vi "test-pose3d.vi"(8 "error in (no error)":errorcluster) -> (0 "error out":errorcluster, 3 "All PASSED":bool)   [LabVIEW 2019]
uses:
  <vilib>/Rock Robotics/WPI/ThirdParty/JAS_Junk/TrajLib/Rotation2d_CreateAngle.vi
  <vilib>/Rock Robotics/WPI/ThirdParty/JAS_Junk/TrajLib/Translation2d_Create.vi
  <vilib>/Rock Robotics/WPI/ThirdParty/JAS_Junk/TrajLib/Quaternion_New.vi
  <vilib>/Rock Robotics/WPI/ThirdParty/JAS_Junk/TrajLib/Pose3d_getTranslation3d.vi
  <vilib>/Rock Robotics/WPI/ThirdParty/JAS_Junk/TrajLib/Translation3d_ToTranslation2d.vi
  <vilib>/Rock Robotics/WPI/ThirdParty/JAS_Junk/TrajLib/Rotation3d_ToRotation2d.vi
  <vilib>/Rock Robotics/WPI/ThirdParty/JAS_Junk/TrajLib/Pose2d_New_TRRO.vi
  <vilib>/Rock Robotics/WPI/ThirdParty/JAS_Junk/TrajLib/Translation2d_Equals.vi
  <vilib>/Rock Robotics/WPI/ThirdParty/JAS_Junk/TrajLib/Rotation2d_Equals.vi
  <vilib>/Rock Robotics/WPI/ThirdParty/JAS_Junk/TrajLib/Matrix_NormF.vi
  <vilib>/Rock Robotics/WPI/ThirdParty/JAS_Junk/TrajLib/Rotation3d_Create_Default.vi
  <vilib>/Rock Robotics/WPI/ThirdParty/JAS_Junk/TrajLib/Quaternion_Get_All.vi
  <vilib>/Rock Robotics/WPI/ThirdParty/JAS_Junk/TrajLib/Rotation3d_GetQuaterion.vi
  <vilib>/Rock Robotics/WPI/ThirdParty/JAS_Junk/TrajLib/Transform3d_GetTranslation3d.vi
  <vilib>/Rock Robotics/WPI/ThirdParty/JAS_Junk/TrajLib/Translation3d_GetXYZ.vi
  <vilib>/Rock Robotics/WPI/ThirdParty/JAS_Junk/TrajLib/Translation3d_Equals.vi
  <vilib>/Rock Robotics/WPI/ThirdParty/JAS_Junk/TrajLib/Rotation3d_Equals.vi
  <vilib>/Rock Robotics/WPI/ThirdParty/JAS_Junk/TrajLib/Transform3d_Create_Pose3dPose3d.vi
  <vilib>/Rock Robotics/WPI/ThirdParty/JAS_Junk/TrajLib/Pose3d_TransformBy.vi
  <vilib>/Rock Robotics/WPI/ThirdParty/JAS_Junk/TrajLib/Util_CalcDist.vi
  <vilib>/Analysis/_algsub.llb/Matrix Norm.vi
  <vilib>/Analysis/_algsub.llb/Real Matrix Norm.vi
  <vilib>/Rock Robotics/WPI/ThirdParty/JAS_Junk/TrajLib/Quaternion_New_Default.vi
  <vilib>/Rock Robotics/WPI/ThirdParty/JAS_Junk/TrajLib/Quaternion_Equals.vi
  <vilib>/Rock Robotics/WPI/ThirdParty/JAS_Junk/TrajLib/Translation3d_Minus.vi
  <vilib>/Rock Robotics/WPI/ThirdParty/JAS_Junk/TrajLib/Translation3d_RotateBy.vi
  <vilib>/Rock Robotics/WPI/ThirdParty/JAS_Junk/TrajLib/Rotation3d_UnaryMinus.vi
  <vilib>/Rock Robotics/WPI/ThirdParty/JAS_Junk/TrajLib/Rotation3d_Minus.vi
  <vilib>/Rock Robotics/WPI/ThirdParty/JAS_Junk/TrajLib/Translation3d_Plus.vi
  <vilib>/Rock Robotics/WPI/ThirdParty/JAS_Junk/TrajLib/Rotation3d_Plus.vi
  <vilib>/Rock Robotics/WPI/ThirdParty/JAS_Junk/TrajLib/Quaternion_Times.vi
  <vilib>/Rock Robotics/WPI/ThirdParty/JAS_Junk/TrajLib/Quaternion_Inverse.vi
  <vilib>/Rock Robotics/WPI/ThirdParty/JAS_Junk/TrajLib/Rotation3d_Create_Quaternion.vi
  <vilib>/Rock Robotics/WPI/ThirdParty/JAS_Junk/TrajLib/Rotation3d_RotateBy.vi
  <vilib>/Rock Robotics/WPI/ThirdParty/JAS_Junk/TrajLib/Quaternion_Get_LVQuat.vi
  <vilib>/Rock Robotics/WPI/ThirdParty/JAS_Junk/TrajLib/Quaternion_New_LVQuat.vi
  <vilib>/Rock Robotics/WPI/ThirdParty/JAS_Junk/TrajLib/Quaternion_Normalize.vi
  <vilib>/Analysis/Matrix/Numeric/Conversions/Array To Matrix.vi
  <vilib>/Analysis/Matrix/Numeric/Conversions/Array To Matrix - RA.vi
  <vilib>/robotics/Kinematics/Multiply Quaternions.vi
  <vilib>/robotics/Kinematics/Multiply Quaternion by Quaternion.vi
  <vilib>/Rock Robotics/WPI/ThirdParty/JAS_Junk/TrajLib/Trajectory_Library.lvlib
panel:
  # "Pose 3D test"
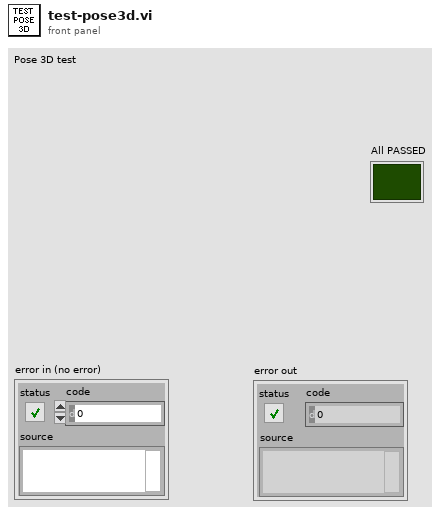
[diagram p1: front panel]
types:
  T1 = typedef "Trajectory_Library.lvlib/TRANSLATION3D.ctl" = cluster{"X":dbl, "Y":dbl, "Z":dbl}
  T2 = typedef "Trajectory_Library.lvlib/ROTATION3D.ctl" = cluster{"Q_quaternion":T3}
  T3 = typedef "Trajectory_Library.lvlib/QUATERNION.ctl" = cluster{"R":dbl, "V":dbl[]}
  T4 = typedef "Trajectory_Library.lvlib/TRANSFORM3D.ctl" = cluster{"TRANSLATION3D":T1, "ROTATION3D":T2}
  T5 = typedef "Trajectory_Library.lvlib/POSE3D.ctl" = cluster{"Translation3d":T1, "Rotation3d":T2}
  T6 = typedef "Trajectory_Library.lvlib/POSE2D.ctl" = cluster{"TRANSLATION":T7, "ROTATION":T8}
  T7 = typedef "Trajectory_Library.lvlib/TRANSLATION2D.ctl" = cluster{"X":dbl, "Y":dbl}
  T8 = typedef "Trajectory_Library.lvlib/ROTATION2D.ctl" = cluster{"VALUE":dbl, "COS":dbl, "SIN":dbl}
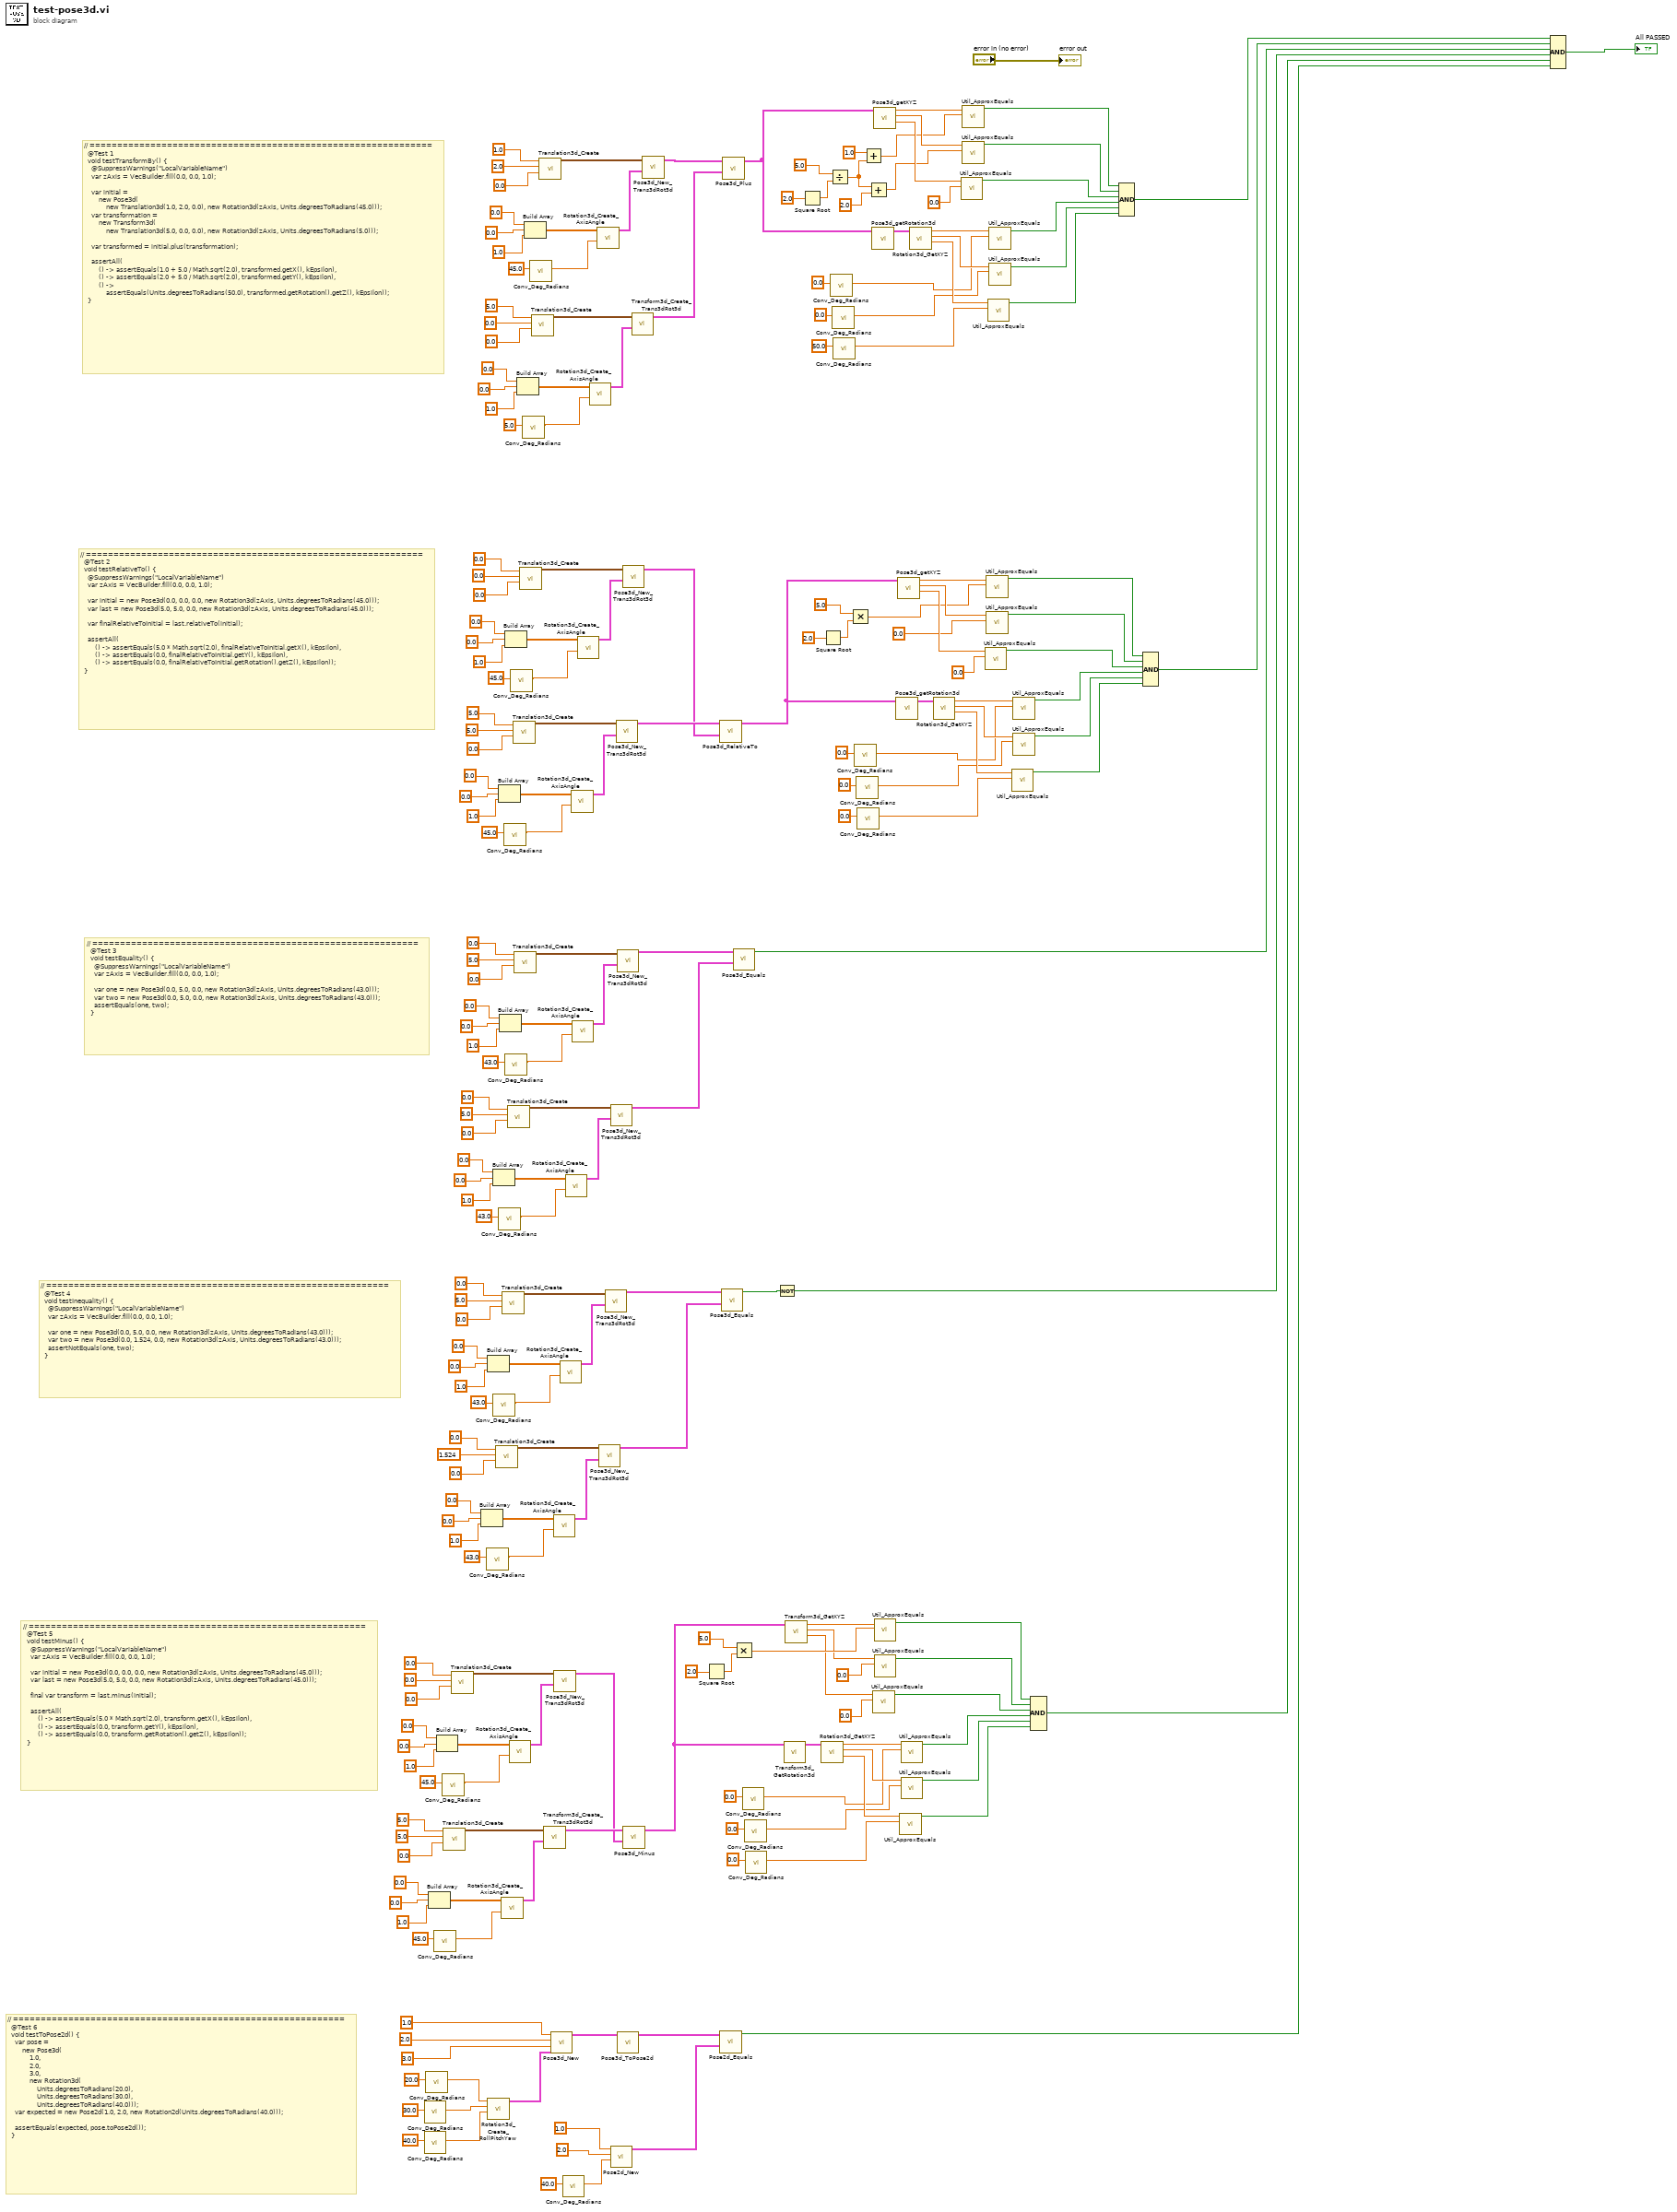
[diagram p0: block diagram]
diagram:
  # "// ============================================================\n  @Test 6\n  void testToPose2d() {\n    var pose =\n        new Pose3d(\n            1.0,\n            2.0,\n            3.0,\n            new Rotation3d(\n                Units.degreesToRadians(20.0),\n                Units.degreesToRadians(30.0),\n                Units.degreesToRadians(40.0)));\n    var expected = new Pose2d(1.0, 2.0, new Rotation2d(Units.degreesToRadians(40.0)));\n\n    assertEquals(expected, pose.toPose2d());\n  }"
  # "// =============================================================\n  @Test 5\n  void testMinus() {\n    @SuppressWarnings(\"LocalVariableName\")\n    var zAxis = VecBuilder.fill(0.0, 0.0, 1.0);\n\n    var initial = new Pose3d(0.0, 0.0, 0.0, new Rotation3d(zAxis, Units.degreesToRadians(45.0)));\n    var last = new Pose3d(5.0, 5.0, 0.0, new Rotation3d(zAxis, Units.degreesToRadians(45.0)));\n\n    final var transform = last.minus(initial);\n\n    assertAll(\n        () -> assertEquals(5.0 * Math.sqrt(2.0), transform.getX(), kEpsilon),\n        () -> assertEquals(0.0, transform.getY(), kEpsilon),\n        () -> assertEquals(0.0, transform.getRotation().getZ(), kEpsilon));\n  }"
  # "// ==============================================================\n  @Test 4\n  void testInequality() {\n    @SuppressWarnings(\"LocalVariableName\")\n    var zAxis = VecBuilder.fill(0.0, 0.0, 1.0);\n\n    var one = new Pose3d(0.0, 5.0, 0.0, new Rotation3d(zAxis, Units.degreesToRadians(43.0)));\n    var two = new Pose3d(0.0, 1.524, 0.0, new Rotation3d(zAxis, Units.degreesToRadians(43.0)));\n    assertNotEquals(one, two);\n  }"
  # "// ===========================================================\n  @Test 3\n  void testEquality() {\n    @SuppressWarnings(\"LocalVariableName\")\n    var zAxis = VecBuilder.fill(0.0, 0.0, 1.0);\n\n    var one = new Pose3d(0.0, 5.0, 0.0, new Rotation3d(zAxis, Units.degreesToRadians(43.0)));\n    var two = new Pose3d(0.0, 5.0, 0.0, new Rotation3d(zAxis, Units.degreesToRadians(43.0)));\n    assertEquals(one, two);\n  }"
  # "// =============================================================\n  @Test 2\n  void testRelativeTo() {\n    @SuppressWarnings(\"LocalVariableName\")\n    var zAxis = VecBuilder.fill(0.0, 0.0, 1.0);\n\n    var initial = new Pose3d(0.0, 0.0, 0.0, new Rotation3d(zAxis, Units.degreesToRadians(45.0)));\n    var last = new Pose3d(5.0, 5.0, 0.0, new Rotation3d(zAxis, Units.degreesToRadians(45.0)));\n\n    var finalRelativeToInitial = last.relativeTo(initial);\n\n    assertAll(\n        () -> assertEquals(5.0 * Math.sqrt(2.0), finalRelativeToInitial.getX(), kEpsilon),\n        () -> assertEquals(0.0, finalRelativeToInitial.getY(), kEpsilon),\n        () -> assertEquals(0.0, finalRelativeToInitial.getRotation().getZ(), kEpsilon));\n  }"
  # "// ==============================================================\n  @Test 1\n  void testTransformBy() {\n    @SuppressWarnings(\"LocalVariableName\")\n    var zAxis = VecBuilder.fill(0.0, 0.0, 1.0);\n\n    var initial =\n        new Pose3d(\n            new Translation3d(1.0, 2.0, 0.0), new Rotation3d(zAxis, Units.degreesToRadians(45.0)));\n    var transformation =\n        new Transform3d(\n            new Translation3d(5.0, 0.0, 0.0), new Rotation3d(zAxis, Units.degreesToRadians(5.0)));\n\n    var transformed = initial.plus(transformation);\n\n    assertAll(\n        () -> assertEquals(1.0 + 5.0 / Math.sqrt(2.0), transformed.getX(), kEpsilon),\n        () -> assertEquals(2.0 + 5.0 / Math.sqrt(2.0), transformed.getY(), kEpsilon),\n        () ->\n            assertEquals(Units.degreesToRadians(50.0), transformed.getRotation().getZ(), kEpsilon));\n  }"
  n1 = call <vilib>:"Conv_Deg_Radians.vi"("Degress"=30.0) -> ("Radians"=w11:dbl)  [unwired: 10 in]
  n2 = call <vilib>:"Conv_Deg_Radians.vi"("Degress"=40.0) -> ("Radians"=w10:dbl)  [unwired: 10 in]
  n3 = call <vilib>:"Conv_Deg_Radians.vi"("Degress"=20.0) -> ("Radians"=w12:dbl)  [unwired: 10 in]
  n4 = Build Array(0.0 ("element"), 0.0 ("element"), 1.0 ("element")) -> (w58:dbl[])
  n5 = call <vilib>:"Conv_Deg_Radians.vi"("Degress"=45.0) -> ("Radians"=w56:dbl)  [unwired: 10 in]
  n6 = Build Array(0.0 ("element"), 0.0 ("element"), 1.0 ("element")) -> (w69:dbl[])
  n7 = call <vilib>:"Conv_Deg_Radians.vi"("Degress"=45.0) -> ("Radians"=w67:dbl)  [unwired: 10 in]
  n8 = call <vilib>:"Translation3d_Create.vi"("Z"=0.0, "Y"=5.0, "X"=5.0) -> ("TRANSLATION3D"=w49:T1)  [unwired: 8 in]
  n9 = call <vilib>:"Translation3d_Create.vi"("Z"=0.0, "Y"=0.0, "X"=0.0) -> ("TRANSLATION3D"=w60:T1)  [unwired: 8 in]
  n10 = Build Array(0.0 ("element"), 0.0 ("element"), 1.0 ("element")) -> (w84:dbl[])
  n11 = call <vilib>:"Conv_Deg_Radians.vi"("Degress"=43.0) -> ("Radians"=w82:dbl)  [unwired: 10 in]
  n12 = Build Array(0.0 ("element"), 0.0 ("element"), 1.0 ("element")) -> (w95:dbl[])
  n13 = call <vilib>:"Rotation3d_Create_RollPitchYaw.vi"("Yaw"=w10, "Pitch"=w11, "Roll"=w12) -> ("Rotation3d"=w9:T2)  [unwired: 8 in]
  n14 = Build Array(0.0 ("element"), 0.0 ("element"), 1.0 ("element")) -> (w109:dbl[])
  n15 = call <vilib>:"Conv_Deg_Radians.vi"("Degress"=43.0) -> ("Radians"=w93:dbl)  [unwired: 10 in]
  n16 = call <vilib>:"Translation3d_Create.vi"("Z"=0.0, "Y"=1.524, "X"=0.0) -> ("TRANSLATION3D"=w75:T1)  [unwired: 8 in]
  n17 = Build Array(0.0 ("element"), 0.0 ("element"), 1.0 ("element")) -> (w160:dbl[])
  n18 = call <vilib>:"Conv_Deg_Radians.vi"("Degress"=43.0) -> ("Radians"=w107:dbl)  [unwired: 10 in]
  n19 = Build Array(0.0 ("element"), 0.0 ("element"), 1.0 ("element")) -> (w120:dbl[])
  n20 = call <vilib>:"Rotation3d_Create_AxisAngle.vi"("Angle"=w56, "Axis Vector"=w58) -> ("Rotation3d"=w48:T2)  [unwired: 9 in]
  n21 = call <vilib>:"Translation3d_Create.vi"("Z"=0.0, "Y"=5.0, "X"=0.0) -> ("TRANSLATION3D"=w86:T1)  [unwired: 8 in]
  n22 = call <vilib>:"Conv_Deg_Radians.vi"("Degress"=45.0) -> ("Radians"=w158:dbl)  [unwired: 10 in]
  n23 = Build Array(0.0 ("element"), 0.0 ("element"), 1.0 ("element")) -> (w171:dbl[])
  n24 = call <vilib>:"Conv_Deg_Radians.vi"("Degress"=43.0) -> ("Radians"=w118:dbl)  [unwired: 10 in]
  n25 = call <vilib>:"Translation3d_Create.vi"("Z"=0.0, "Y"=5.0, "X"=0.0) -> ("TRANSLATION3D"=w100:T1)  [unwired: 8 in]
  n26 = call <vilib>:"Rotation3d_Create_AxisAngle.vi"("Angle"=w67, "Axis Vector"=w69) -> ("Rotation3d"=w59:T2)  [unwired: 9 in]
  n27 = call <vilib>:"Conv_Deg_Radians.vi"("Degress"=45.0) -> ("Radians"=w169:dbl)  [unwired: 10 in]
  n28 = call <vilib>:"Translation3d_Create.vi"("Z"=0.0, "Y"=5.0, "X"=5.0) -> ("TRANSLATION3D"=w151:T1)  [unwired: 8 in]
  n29 = call <vilib>:"Translation3d_Create.vi"("Z"=0.0, "Y"=5.0, "X"=0.0) -> ("TRANSLATION3D"=w111:T1)  [unwired: 8 in]
  n30 = Build Array(0.0 ("element"), 0.0 ("element"), 1.0 ("element")) -> (w215:dbl[])
  n31 = call <vilib>:"Translation3d_Create.vi"("Z"=0.0, "Y"=0.0, "X"=0.0) -> ("TRANSLATION3D"=w162:T1)  [unwired: 8 in]
  n32 = call <vilib>:"Conv_Deg_Radians.vi"("Degress"=5.0) -> ("Radians"=w213:dbl)  [unwired: 10 in]
  n33 = Build Array(0.0 ("element"), 0.0 ("element"), 1.0 ("element")) -> (w226:dbl[])
  n34 = call <vilib>:"Conv_Deg_Radians.vi"("Degress"=45.0) -> ("Radians"=w224:dbl)  [unwired: 10 in]
  n35 = call <vilib>:"Translation3d_Create.vi"("Z"=0.0, "Y"=0.0, "X"=5.0) -> ("TRANSLATION3D"=w206:T1)  [unwired: 8 in]
  n36 = call <vilib>:"Translation3d_Create.vi"("Z"=0.0, "Y"=2.0, "X"=1.0) -> ("TRANSLATION3D"=w217:T1)  [unwired: 8 in]
  n37 = call <vilib>:"Transform3d_Create_Trans3dRot3d.vi"("Rotation3d"=w48, "Translation3d"=w49) -> ("Transform3d"=w21:T4)  [unwired: 9 in]
  n38 = call <vilib>:"Pose3d_New.vi"("Rotation3d"=w9, "z"=3.0 ("Z"), "Y"=2.0, "X"=1.0) -> ("out Pose3d"=w8:T5)  [unwired: 7 in]
  n39 = call <vilib>:"Rotation3d_Create_AxisAngle.vi"("Angle"=w82, "Axis Vector"=w84) -> ("Rotation3d"=w74:T2)  [unwired: 9 in]
  n40 = call <vilib>:"Pose3d_New_Trans3dRot3d.vi"("Rotation3d"=w59, "Translation3d"=w60) -> ("outPose3d"=w20:T5)  [unwired: 9 in]
  n41 = call <vilib>:"Rotation3d_Create_AxisAngle.vi"("Angle"=w93, "Axis Vector"=w95) -> ("Rotation3d"=w85:T2)  [unwired: 9 in]
  n42 = call <vilib>:"Conv_Deg_Radians.vi"("Degress"=40.0) -> ("Radians"=w4:dbl)  [unwired: 10 in]
  n43 = call <vilib>:"Rotation3d_Create_AxisAngle.vi"("Angle"=w107, "Axis Vector"=w109) -> ("Rotation3d"=w99:T2)  [unwired: 9 in]
  n44 = call <vilib>:"Rotation3d_Create_AxisAngle.vi"("Angle"=w158, "Axis Vector"=w160) -> ("Rotation3d"=w150:T2)  [unwired: 9 in]
  n45 = call <vilib>:"Rotation3d_Create_AxisAngle.vi"("Angle"=w118, "Axis Vector"=w120) -> ("Rotation3d"=w110:T2)  [unwired: 9 in]
  n46 = call <vilib>:"Rotation3d_Create_AxisAngle.vi"("Angle"=w169, "Axis Vector"=w171) -> ("Rotation3d"=w161:T2)  [unwired: 9 in]
  n47 = call <vilib>:"Rotation3d_Create_AxisAngle.vi"("Angle"=w213, "Axis Vector"=w215) -> ("Rotation3d"=w205:T2)  [unwired: 9 in]
  n48 = call <vilib>:"Rotation3d_Create_AxisAngle.vi"("Angle"=w224, "Axis Vector"=w226) -> ("Rotation3d"=w216:T2)  [unwired: 9 in]
  n49 = call <vilib>:"Pose3d_New_Trans3dRot3d.vi"("Rotation3d"=w74, "Translation3d"=w75) -> ("outPose3d"=w72:T5)  [unwired: 9 in]
  n50 = call <vilib>:"Pose3d_New_Trans3dRot3d.vi"("Rotation3d"=w85, "Translation3d"=w86) -> ("outPose3d"=w73:T5)  [unwired: 9 in]
  n51 = call <vilib>:"Pose3d_New_Trans3dRot3d.vi"("Rotation3d"=w99, "Translation3d"=w100) -> ("outPose3d"=w97:T5)  [unwired: 9 in]
  n52 = call <vilib>:"Pose2d_New.vi"("Heading"=w4, "Y"=2.0 ("X"), "X"=1.0) -> ("out POSe"=w2:T6)  [unwired: 8 in]
  n53 = call <vilib>:"Pose3d_New_Trans3dRot3d.vi"("Rotation3d"=w150, "Translation3d"=w151) -> ("outPose3d"=w149:T5)  [unwired: 9 in]
  n54 = call <vilib>:"Pose3d_New_Trans3dRot3d.vi"("Rotation3d"=w110, "Translation3d"=w111) -> ("outPose3d"=w98:T5)  [unwired: 9 in]
  n55 = call <vilib>:"Pose3d_ToPose2d.vi"("in Pose3d"=w8) -> ("out Pose2d"=w3:T6)  [unwired: 10 in]
  n56 = call <vilib>:"Pose3d_New_Trans3dRot3d.vi"("Rotation3d"=w161, "Translation3d"=w162) -> ("outPose3d"=w148:T5)  [unwired: 9 in]
  n57 = call <vilib>:"Pose3d_Minus.vi"("other Transform3d"=w20, "in Pose3d"=w21) -> ("outTransform3d"=w36:T4)  [unwired: 9 in]
  n58 = call <vilib>:"Transform3d_Create_Trans3dRot3d.vi"("Rotation3d"=w205, "Translation3d"=w206) -> ("Transform3d"=w190:T4)  [unwired: 9 in]
  n59 = call <vilib>:"Pose3d_New_Trans3dRot3d.vi"("Rotation3d"=w216, "Translation3d"=w217) -> ("outPose3d"=w191:T5)  [unwired: 9 in]
  n60 = Square Root(x=2.0) -> (sqrt(x)=w33:dbl)
  n61 = call <vilib>:"Pose3d_RelativeTo.vi"("other Pose3d"=w148, "in Pose3d"=w149) -> ("out Pose3d"=w124:T5)  [unwired: 9 in]
  n62 = call <vilib>:"Pose2d_Equals.vi"("other POSE"=w2, "in POSE"=w3) -> ("Equals"=w1:bool)  [unwired: 9 in]
  n63 = call <vilib>:"Pose3d_Equals.vi"("other Pose3d"=w72, "in Pose3d"=w73) -> ("Equals"=w71:bool)  [unwired: 9 in]
  n64 = call <vilib>:"Pose3d_Plus.vi"("other Transform3d"=w190, "in Pose3d"=w191) -> ("out Pose3d"=w189:T5)  [unwired: 9 in]
  n65 = call <vilib>:"Pose3d_Equals.vi"("other Pose3d"=w97, "in Pose3d"=w98) -> ("Equals"=w96:bool)  [unwired: 9 in]
  n66 = Multiply(x=5.0, y=w33) -> (x*y=w25:dbl)
  n67 = call <vilib>:"Conv_Deg_Radians.vi"("Degress"=0.0) -> ("Radians"=w26:dbl)  [unwired: 10 in]
  n68 = call <vilib>:"Conv_Deg_Radians.vi"("Degress"=0.0) -> ("Radians"=w27:dbl)  [unwired: 10 in]
  n69 = call <vilib>:"Conv_Deg_Radians.vi"("Degress"=0.0) -> ("Radians"=w28:dbl)  [unwired: 10 in]
  n70 = Not(x=w71) -> (.not. x?=w70:bool)
  n71 = call <vilib>:"Transform3d_GetRotation3d.vi"("in Transform3d"=w36) -> ("Rotation3d"=w46:T2)  [unwired: 10 in]
  n72 = call <vilib>:"Transform3d_GetXYZ.vi"("inTransform3d"=w36) -> ("Z"=w22:dbl, "Y"=w23:dbl, "X"=w47:dbl)  [unwired: 8 in]
  n73 = Square Root(x=2.0) -> (sqrt(x)=w186:dbl)
  n74 = call <vilib>:"Rotation3d_GetXYZ.vi"("in Rotation3d"=w46) -> ("Z"=w43:dbl, "Y"=w44:dbl, "X"=w45:dbl)  [unwired: 8 in]
  n75 = Square Root(x=2.0) -> (sqrt(x)=w132:dbl)
  n76 = Divide(x=5.0, y=w186) -> (x/y=w183:dbl)
  n77 = call <vilib>:"Conv_Deg_Radians.vi"("Degress"=0.0) -> ("Radians"=w174:dbl)  [unwired: 10 in]
  n78 = call <vilib>:"Conv_Deg_Radians.vi"("Degress"=0.0) -> ("Radians"=w175:dbl)  [unwired: 10 in]
  n79 = call <vilib>:"Conv_Deg_Radians.vi"("Degress"=50.0) -> ("Radians"=w176:dbl)  [unwired: 10 in]
  n80 = Multiply(x=5.0, y=w132) -> (x*y=w123:dbl)
  n81 = call <vilib>:"Conv_Deg_Radians.vi"("Degress"=0.0) -> ("Radians"=w125:dbl)  [unwired: 10 in]
  n82 = call <vilib>:"Conv_Deg_Radians.vi"("Degress"=0.0) -> ("Radians"=w126:dbl)  [unwired: 10 in]
  n83 = call <vilib>:"Conv_Deg_Radians.vi"("Degress"=0.0) -> ("Radians"=w127:dbl)  [unwired: 10 in]
  n84 = Add(x=1.0, y=w183) -> (x+y=w185:dbl)
  n85 = Add(x=w183, y=2.0) -> (x+y=w184:dbl)
  n86 = call <vilib>:"Pose3d_getRotation3d.vi"("in Pose3d"=w189) -> ("out Rotation3d"=w201:T2)  [unwired: 10 in]
  n87 = call <vilib>:"Util_ApproxEquals.vi"("Value 2"=0.0, "Value 1"=w22) -> ("ApproxEquals"=w40:bool)  [unwired: 9 in]
  n88 = call <vilib>:"Pose3d_getXYZ.vi"("in Pose3d"=w189) -> ("Z"=w202:dbl, "Y"=w203:dbl, "X"=w204:dbl)  [unwired: 8 in]
  n89 = call <vilib>:"Util_ApproxEquals.vi"("Value 2"=w25, "Value 1"=w47) -> ("ApproxEquals"=w42:bool)  [unwired: 9 in]
  n90 = call <vilib>:"Util_ApproxEquals.vi"("Value 2"=0.0, "Value 1"=w23) -> ("ApproxEquals"=w41:bool)  [unwired: 9 in]
  n91 = call <vilib>:"Pose3d_getRotation3d.vi"("in Pose3d"=w124) -> ("out Rotation3d"=w144:T2)  [unwired: 10 in]
  n92 = call <vilib>:"Pose3d_getXYZ.vi"("in Pose3d"=w124) -> ("Z"=w145:dbl, "Y"=w146:dbl, "X"=w147:dbl)  [unwired: 8 in]
  n93 = call <vilib>:"Util_ApproxEquals.vi"("Value 2"=w28, "Value 1"=w43) -> ("ApproxEquals"=w37:bool)  [unwired: 9 in]
  n94 = call <vilib>:"Util_ApproxEquals.vi"("Value 2"=w26, "Value 1"=w45) -> ("ApproxEquals"=w39:bool)  [unwired: 9 in]
  n95 = call <vilib>:"Util_ApproxEquals.vi"("Value 2"=w27, "Value 1"=w44) -> ("ApproxEquals"=w38:bool)  [unwired: 9 in]
  n96 = call <vilib>:"Rotation3d_GetXYZ.vi"("in Rotation3d"=w201) -> ("Z"=w198:dbl, "Y"=w199:dbl, "X"=w200:dbl)  [unwired: 8 in]
  n97 = call <vilib>:"Rotation3d_GetXYZ.vi"("in Rotation3d"=w144) -> ("Z"=w141:dbl, "Y"=w142:dbl, "X"=w143:dbl)  [unwired: 8 in]
  n98 = call <vilib>:"Util_ApproxEquals.vi"("Value 2"=0.0, "Value 1"=w202) -> ("ApproxEquals"=w195:bool)  [unwired: 9 in]
  n99 = call <vilib>:"Util_ApproxEquals.vi"("Value 2"=w185, "Value 1"=w204) -> ("ApproxEquals"=w197:bool)  [unwired: 9 in]
  n100 = call <vilib>:"Util_ApproxEquals.vi"("Value 2"=w184, "Value 1"=w203) -> ("ApproxEquals"=w196:bool)  [unwired: 9 in]
  n101 = call <vilib>:"Util_ApproxEquals.vi"("Value 2"=0.0, "Value 1"=w145) -> ("ApproxEquals"=w138:bool)  [unwired: 9 in]
  n102 = call <vilib>:"Util_ApproxEquals.vi"("Value 2"=w123, "Value 1"=w147) -> ("ApproxEquals"=w140:bool)  [unwired: 9 in]
  n103 = call <vilib>:"Util_ApproxEquals.vi"("Value 2"=0.0, "Value 1"=w146) -> ("ApproxEquals"=w139:bool)  [unwired: 9 in]
  n104 = call <vilib>:"Util_ApproxEquals.vi"("Value 2"=w176, "Value 1"=w198) -> ("ApproxEquals"=w192:bool)  [unwired: 9 in]
  n105 = call <vilib>:"Util_ApproxEquals.vi"("Value 2"=w174, "Value 1"=w200) -> ("ApproxEquals"=w194:bool)  [unwired: 9 in]
  n106 = call <vilib>:"Util_ApproxEquals.vi"("Value 2"=w175, "Value 1"=w199) -> ("ApproxEquals"=w193:bool)  [unwired: 9 in]
  n107 = call <vilib>:"Util_ApproxEquals.vi"("Value 2"=w127, "Value 1"=w141) -> ("ApproxEquals"=w135:bool)  [unwired: 9 in]
  n108 = call <vilib>:"Util_ApproxEquals.vi"("Value 2"=w125, "Value 1"=w143) -> ("ApproxEquals"=w137:bool)  [unwired: 9 in]
  n109 = call <vilib>:"Util_ApproxEquals.vi"("Value 2"=w126, "Value 1"=w142) -> ("ApproxEquals"=w136:bool)  [unwired: 9 in]
  n110 = Compound Arithmetic op=AND(w42, w41, w40, w39, w38, w37) -> (w24:bool)
  n111 = Compound Arithmetic op=AND(w197, w196, w195, w194, w193, w192) -> (w172:bool)
  n112 = Compound Arithmetic op=AND(w140, w139, w138, w137, w136, w135) -> (w121:bool)
  n113 = Compound Arithmetic op=AND(w172, w121, w96, w70, w24, w1) -> (→"All PASSED":bool)
  "error out" <- "error in (no error)"
